vi "Load vs time.vi"(1 "Reset":bool) -> (8 "Time(s)":dbl)   [LabVIEW 2017]
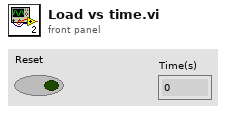
[diagram p1: front panel]
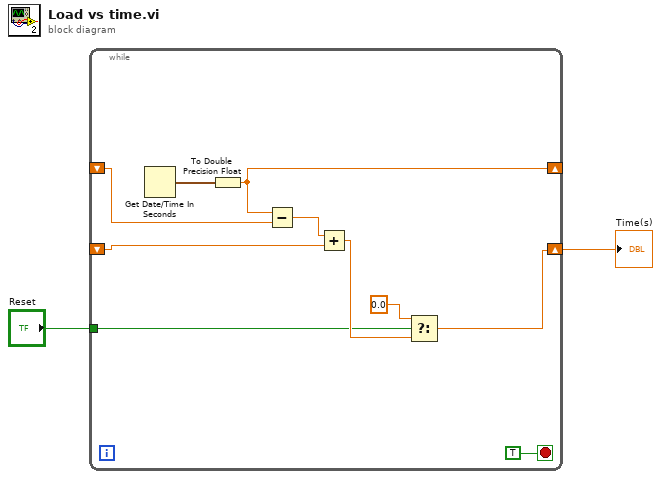
[diagram p0: block diagram]
diagram:
  n1 = while {
    shift-right: [w10] -> _
    shift-left: _ -> [w11]
    shift-right: [w3] -> w2
    shift-left: _ -> [w8]
    tunnel: "Reset" -> [w4]
    stop <- TRUE stop-if-true
    n2 = Get Date/Time In Seconds() -> (seconds since 1Jan1904=w12:timestamp)
    n3 = To Double Precision Float(number=w12) -> (double precision float=w10:dbl)
    n4 = Subtract(x=w10, y=w11) -> (x-y=w9:dbl)
    n5 = Add(x=w9, y=w8) -> (x+y=w6:dbl)
    n6 = Select(t=0.0, s=w4, f=w6) -> (s? t:f=w3:dbl)
  }
  "Time(s)" <- w2
